vi "Get Read Speeds.vi"(8 "error in (no error)":errorcluster, 10 "camera model":string, 11 "Handle in":u32) -> (0 "error out":errorcluster, 2 "Readout Times (s)":dbl[](array[numeric]), 3 "Handle out":u32)   [LabVIEW 2023, in "Hamamatsu Camera.lvlib"]
uses:
  Hamamatsu Camera.lvlib
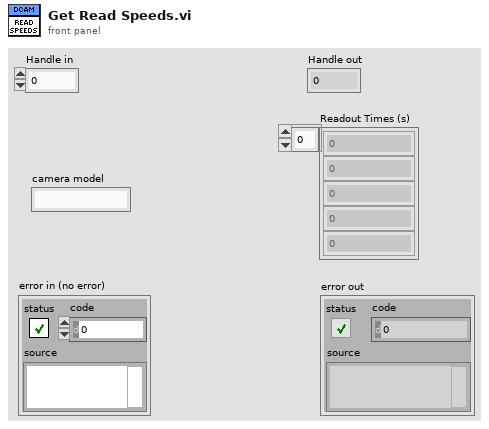
[diagram p1: front panel]
types:
  T1 = cluster{"Range":cluster{"min":dbl, "max":dbl, "step":dbl}, "default":dbl, "views":u32, "Writable":bool, "Text Values":bool, "Value Names":cluster{"Name":string, "Value":dbl}[]}
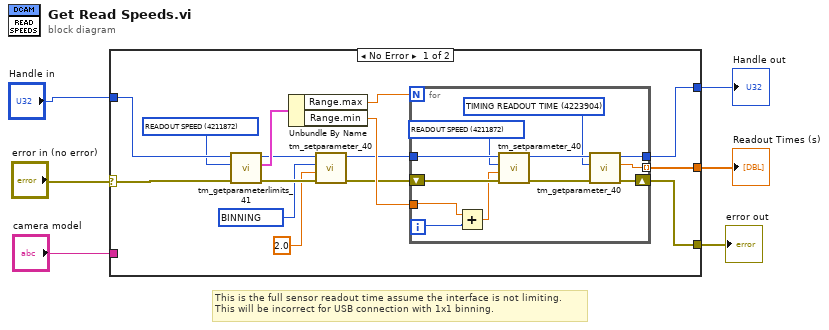
[diagram p0: block diagram]
diagram:
  # "This is the full sensor readout time assume the interface is not limiting.\nThis will be incorrect for USB connection with 1x1 binning."
  n1 = case shown="No Error" "error in (no error)" {
    selector: "error in (no error)" -> [w17 w34]
    tunnel: [w21 _] -> w6
    tunnel: [w20 w35] -> w5
    tunnel: [w19 w34] -> w4
    tunnel: "Handle in" -> [w18 w35]
    tunnel: "camera model" -> [_ _]
    frame No Error {
      w8 = u32 4215968 items=["SENSOR MODE"=4212128, "READOUT SPEED"=4211872, "BIT PER CHANNEL"=4342976, "TRIGGER SOURCE"=1066144, "TRIGGER MODE"=1066400, "TRIGGER ACTIVE"=1066160, "TRIGGER GLOBAL EXPOSURE"=2049680, "TRIGGER POLARITY"=1066416, "TRIGGER DELAY"=1066480, "SENSOR COOLER STATUS"=2115280, "EXPOSURE TIME CONTROL"=2049216, "EXPOSURE TIME"=2049184, "DEFECT CORRECT MODE"=4670368, "BINNING"=4215968, "TIMING READOUT TIME"=4223904, "INTERNAL FRAME RATE"=4225952, "INTERNAL FRAME INTERVAL"=4225968, "IMAGE WIDTH"=4343200, "IMAGE HEIGHT"=4343216, "IMAGE ROWBYTES"=4343232, "IMAGE FRAMEBYTES"=4343248, "IMAGE PIXEL TYPE"=4343296, "NUMBER OF OUTPUT TRIGGER CONNECTOR"=1852320, "OUTPUT TRIGGER SOURCE[0]"=1852576, "OUTPUT TRIGGER SOURCE[1]"=1852832, "OUTPUT TRIGGER SOURCE[2]"=1853088, "OUTPUT TRIGGER POLARITY[0]"=1852592, "OUTPUT TRIGGER POLARITY[1]"=1852848, "OUTPUT TRIGGER POLARITY[2]"=1853104, "OUTPUT TRIGGER ACTIVE[0]"=1852608, "OUTPUT TRIGGER ACTIVE[1]"=1852864, "OUTPUT TRIGGER ACTIVE[2]"=1853120, "OUTPUT TRIGGER DELAY[0]"=1852624, "OUTPUT TRIGGER DELAY[1]"=1852880, "OUTPUT TRIGGER DELAY[2]"=1853136, "OUTPUT TRIGGER PERIOD[0]"=1852640, "OUTPUT TRIGGER PERIOD[1]"=1852896, "OUTPUT TRIGGER PERIOD[2]"=1853152, "OUTPUT TRIGGER KIND[0]"=1852656, "OUTPUT TRIGGER KIND[1]"=1852912, "OUTPUT TRIGGER KIND[2]"=1853168] ("Parameter")
      w13 = u32 4211872 items=["SENSOR MODE"=4212128, "READOUT SPEED"=4211872, "READOUT DIRECTION"=4211904, "BIT PER CHANNEL"=4342976, "TRIGGER SOURCE"=1066144, "TRIGGER MODE"=1066400, "TRIGGER ACTIVE"=1066160, "TRIGGER GLOBAL EXPOSURE"=2049680, "TRIGGER POLARITY"=1066416, "TRIGGER CONNECTOR"=1066432, "TRIGGER DELAY"=1066480, "SENSOR TEMPERATURE"=2115232, "SENSOR COOLER STATUS"=2115280, "EXPOSURE TIME"=2049184, "DEFECT CORRECT MODE"=4670368, "HOT PIXEL CORRECT LEVEL"=4670400, "BINNING"=4215968, "TIMING READOUT TIME"=4223904, "INTERNAL FRAME RATE"=4225952, "INTERNAL FRAME INTERVAL"=4225968, "INTERNAL LINE SPEED"=4226000, "INTERNAL LINE INTERVAL"=4226016, "IMAGE WIDTH"=4343200, "IMAGE HEIGHT"=4343216, "IMAGE ROWBYTES"=4343232, "IMAGE FRAMEBYTES"=4343248, "IMAGE PIXEL TYPE"=4343296, "NUMBER OF OUTPUT TRIGGER CONNECTOR"=1852320, "OUTPUT TRIGGER SOURCE[0]"=1852576, "OUTPUT TRIGGER SOURCE[1]"=1852832, "OUTPUT TRIGGER SOURCE[2]"=1853088, "OUTPUT TRIGGER POLARITY[0]"=1852592, "OUTPUT TRIGGER POLARITY[1]"=1852848, "OUTPUT TRIGGER POLARITY[2]"=1853104, "OUTPUT TRIGGER ACTIVE[0]"=1852608, "OUTPUT TRIGGER ACTIVE[1]"=1852864, "OUTPUT TRIGGER ACTIVE[2]"=1853120, "OUTPUT TRIGGER DELAY[0]"=1852624, "OUTPUT TRIGGER DELAY[1]"=1852880, "OUTPUT TRIGGER DELAY[2]"=1853136, "OUTPUT TRIGGER PERIOD[0]"=1852640, "OUTPUT TRIGGER PERIOD[1]"=1852896, "OUTPUT TRIGGER PERIOD[2]"=1853152, "OUTPUT TRIGGER KIND[0]"=1852656, "OUTPUT TRIGGER KIND[1]"=1852912, "OUTPUT TRIGGER KIND[2]"=1853168, "OUTPUT TRIGGER PRE HSYNC COUNT"=1852704] ("Parameter")
      n2 = call <userlib>:"tm_getparameterlimits_41.vi"("error in (no error)"=w17, "Parameter"=w13, "Handle in"=w18) -> ("error out"=w12:errorcluster, "Limits"=w16:T1, "Handle out"=w11:u32)  [unwired: 6 in]
      n3 = Unbundle By Name(w16) -> ("Range.max"=w14:dbl, "Range.min"=w15:dbl)
      n4 = call <userlib>:"tm_setparameter_40.vi"("error in (no error)"=w12, "Value in"=2.0, "Parameter"=w8, "Handle in"=w11) -> ("error out"=w10:errorcluster, "Handle out"=w9:u32)  [unwired: 6 in]
      n5 = for {
        N: w14 -> [_]
        shift-right: [w25] -> w19
        shift-left: w10 -> [w31]
        tunnel: w9 -> [w30]
        tunnel: w15 -> [w32]
        tunnel: [w24] -> w20
        tunnel: [w23] -> w21 mode=indexing
        i -> [w33]
        w22 = u32 4223904 items=["SENSOR MODE"=4212128, "READOUT SPEED"=4211872, "READOUT DIRECTION"=4211904, "BIT PER CHANNEL"=4342976, "TRIGGER SOURCE"=1066144, "TRIGGER MODE"=1066400, "TRIGGER ACTIVE"=1066160, "TRIGGER GLOBAL EXPOSURE"=2049680, "TRIGGER POLARITY"=1066416, "TRIGGER CONNECTOR"=1066432, "TRIGGER DELAY"=1066480, "SENSOR TEMPERATURE"=2115232, "SENSOR COOLER STATUS"=2115280, "EXPOSURE TIME"=2049184, "DEFECT CORRECT MODE"=4670368, "HOT PIXEL CORRECT LEVEL"=4670400, "BINNING"=4215968, "TIMING READOUT TIME"=4223904, "INTERNAL FRAME RATE"=4225952, "INTERNAL FRAME INTERVAL"=4225968, "INTERNAL LINE SPEED"=4226000, "INTERNAL LINE INTERVAL"=4226016, "IMAGE WIDTH"=4343200, "IMAGE HEIGHT"=4343216, "IMAGE ROWBYTES"=4343232, "IMAGE FRAMEBYTES"=4343248, "IMAGE PIXEL TYPE"=4343296, "NUMBER OF OUTPUT TRIGGER CONNECTOR"=1852320, "OUTPUT TRIGGER SOURCE[0]"=1852576, "OUTPUT TRIGGER SOURCE[1]"=1852832, "OUTPUT TRIGGER SOURCE[2]"=1853088, "OUTPUT TRIGGER POLARITY[0]"=1852592, "OUTPUT TRIGGER POLARITY[1]"=1852848, "OUTPUT TRIGGER POLARITY[2]"=1853104, "OUTPUT TRIGGER ACTIVE[0]"=1852608, "OUTPUT TRIGGER ACTIVE[1]"=1852864, "OUTPUT TRIGGER ACTIVE[2]"=1853120, "OUTPUT TRIGGER DELAY[0]"=1852624, "OUTPUT TRIGGER DELAY[1]"=1852880, "OUTPUT TRIGGER DELAY[2]"=1853136, "OUTPUT TRIGGER PERIOD[0]"=1852640, "OUTPUT TRIGGER PERIOD[1]"=1852896, "OUTPUT TRIGGER PERIOD[2]"=1853152, "OUTPUT TRIGGER KIND[0]"=1852656, "OUTPUT TRIGGER KIND[1]"=1852912, "OUTPUT TRIGGER KIND[2]"=1853168, "OUTPUT TRIGGER PRE HSYNC COUNT"=1852704] ("Parameter")
        w28 = u32 4211872 items=["SENSOR MODE"=4212128, "READOUT SPEED"=4211872, "READOUT DIRECTION"=4211904, "BIT PER CHANNEL"=4342976, "TRIGGER SOURCE"=1066144, "TRIGGER MODE"=1066400, "TRIGGER ACTIVE"=1066160, "TRIGGER GLOBAL EXPOSURE"=2049680, "TRIGGER POLARITY"=1066416, "TRIGGER CONNECTOR"=1066432, "TRIGGER DELAY"=1066480, "SENSOR TEMPERATURE"=2115232, "SENSOR COOLER STATUS"=2115280, "EXPOSURE TIME"=2049184, "DEFECT CORRECT MODE"=4670368, "HOT PIXEL CORRECT LEVEL"=4670400, "BINNING"=4215968, "TIMING READOUT TIME"=4223904, "INTERNAL FRAME RATE"=4225952, "INTERNAL FRAME INTERVAL"=4225968, "INTERNAL LINE SPEED"=4226000, "INTERNAL LINE INTERVAL"=4226016, "IMAGE WIDTH"=4343200, "IMAGE HEIGHT"=4343216, "IMAGE ROWBYTES"=4343232, "IMAGE FRAMEBYTES"=4343248, "IMAGE PIXEL TYPE"=4343296, "NUMBER OF OUTPUT TRIGGER CONNECTOR"=1852320, "OUTPUT TRIGGER SOURCE[0]"=1852576, "OUTPUT TRIGGER SOURCE[1]"=1852832, "OUTPUT TRIGGER SOURCE[2]"=1853088, "OUTPUT TRIGGER POLARITY[0]"=1852592, "OUTPUT TRIGGER POLARITY[1]"=1852848, "OUTPUT TRIGGER POLARITY[2]"=1853104, "OUTPUT TRIGGER ACTIVE[0]"=1852608, "OUTPUT TRIGGER ACTIVE[1]"=1852864, "OUTPUT TRIGGER ACTIVE[2]"=1853120, "OUTPUT TRIGGER DELAY[0]"=1852624, "OUTPUT TRIGGER DELAY[1]"=1852880, "OUTPUT TRIGGER DELAY[2]"=1853136, "OUTPUT TRIGGER PERIOD[0]"=1852640, "OUTPUT TRIGGER PERIOD[1]"=1852896, "OUTPUT TRIGGER PERIOD[2]"=1853152, "OUTPUT TRIGGER KIND[0]"=1852656, "OUTPUT TRIGGER KIND[1]"=1852912, "OUTPUT TRIGGER KIND[2]"=1853168, "OUTPUT TRIGGER PRE HSYNC COUNT"=1852704] ("Parameter")
        n6 = Add(x=w32, y=w33) -> (x+y=w29:dbl)
        n7 = call <userlib>:"tm_setparameter_40.vi"("error in (no error)"=w31, "Value in"=w29, "Parameter"=w28, "Handle in"=w30) -> ("error out"=w26:errorcluster, "Handle out"=w27:u32)  [unwired: 6 in]
        n8 = call <userlib>:"tm_getparameter_40.vi"("error in (no error)"=w26, "Parameter"=w22, "Handle in"=w27) -> ("error out"=w25:errorcluster, "Value out"=w23:dbl, "Handle out"=w24:u32)  [unwired: 6 in]
      }
    }
    frame Error {
    }
  }
  "Readout Times (s)" <- w6
  "Handle out" <- w5
  "error out" <- w4
